vi "Configure Source User Delay.vi"(6 "Delay Time (0 sec)":dbl min=0.0 max=1000.0, 8 "error in (no error)":errorcluster, 9 "User Delay (1)":i32=1 min=1 max=5 step=1, 10 "Function (0: Volts)":u16(ring) items=["Volts", "Current"], 11 "VISA resource name":refnum<visa-resource-name>) -> (0 "error out":errorcluster, 3 "VISA resource name out":refnum<visa-resource-name>)   [LabVIEW 2022 SP3, in "Keithley 2450.lvlib"]
doc: "This VI sets a user-defined delay that can be used in the trigger model."
uses:
  Keithley 2450.lvlib
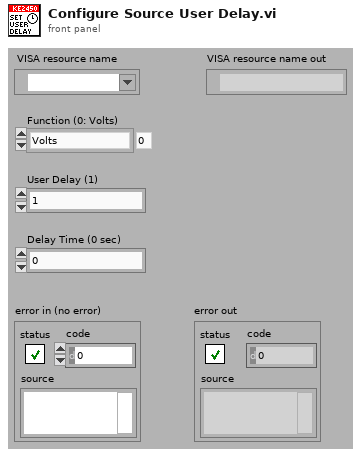
[diagram p1: front panel]
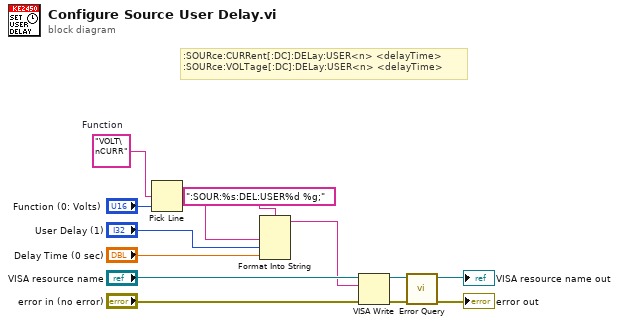
[diagram p0: block diagram]
diagram:
  w5 = "VOLT\nCURR"  # Function
  # ":SOURce:CURRent[:DC]:DELay:USER<n> <delayTime>\n:SOURce:VOLTage[:DC]:DELay:USER<n> <delayTime>"
  n1 = Pick Line(multi-line string=w5, line index="Function (0: Volts)") -> (output string=w3:string)  [unwired: 1 out]
  n2 = Format Into String(format string=":SOUR:%s:DEL:USER%d %g;", w3, "User Delay (1)", "Delay Time (0 sec)") -> (resulting string=w6:string)  [unwired: 2 in, 1 out]
  n3 = VISA Write(VISA resource name="VISA resource name", write buffer=w6, error in (no error)="error in (no error)") -> (VISA resource name out=w11:refnum<visa-resource-name>, error out=w10:errorcluster)  [unwired: 1 out]
  n4 = call "Error Query.vi"("error in (no error)"=w10, "VISA resource name"=w11) -> ("error out"=→"error out":errorcluster, "VISA resource name out"=→"VISA resource name out":refnum<visa-resource-name>)  [unwired: 8 out]
